vi "PAN_Send_InternalCmd.vi"(4 "timeout in ms (-1)":i32=30000, 6 "wait response":bool=TRUE, 7 "taskID":string, 8 "error in (no error)":errorcluster, 10 "command":string) -> (0 "error out":errorcluster, 2 "response":string)   [LabVIEW 2016]
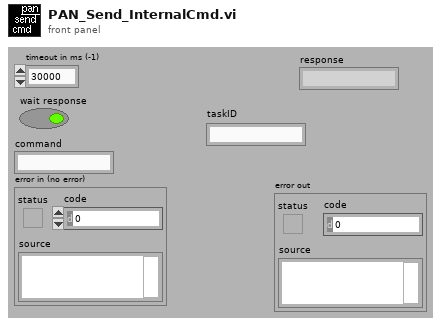
[diagram p1: front panel]
types:
  T1 = typedef "PAN_cmdStruct.ctl" = cluster{"command":string, "resp Q":refnum<queue>}
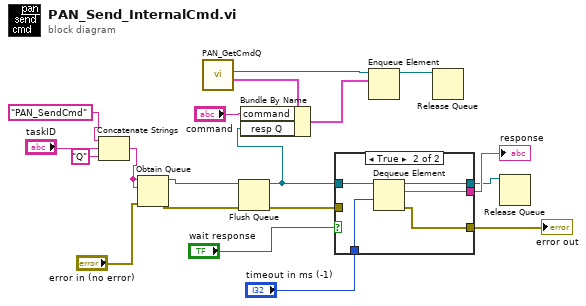
[diagram p0: block diagram]
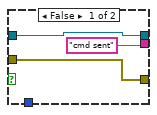
[diagram p2: hidden frame]
diagram:
  n1 = Concatenate Strings("PAN_SendCmd" ("name (unnamed)"), "taskID", "Q" ("string")) -> (w1:string)
  n2 = Obtain Queue(name (unnamed)=w1, element data type=w1, error in (no error)="error in (no error)") -> (queue out=w8:refnum<queue>, error out=w10:errorcluster)  [unwired: 2 in, 1 out]
  n3 = call "PAN_GetCmdQ.vi"() -> ("cmd struct"=w19:T1, "cmdQ"=w18:refnum<queue>)  [unwired: 10 out]
  n4 = Flush Queue(queue=w8, error in (no error)=w10) -> (queue out=w5:refnum<queue>, error out=w11:errorcluster)  [unwired: 1 out]
  n5 = Bundle By Name(cluster=w19, "command"="command", "resp Q"=w5) -> (w17:T1)
  n6 = case shown="True" "wait response" {
    tunnel: w5 -> [w20 w25]
    tunnel: "timeout in ms (-1)" -> [_ w27]
    tunnel: [w22 w26] -> w12
    tunnel: w11 -> [w22 _]
    tunnel: ["cmd sent" ("name (unnamed)") w24] -> w7
    tunnel: [w20 w23] -> w6
    frame False {
    }
    frame True {
      n7 = Dequeue Element(queue=w25, timeout in ms (-1)=w27) -> (queue out=w23:refnum<queue>, element=w24:string, error out=w26:errorcluster)  [unwired: 1 in, 1 out]
    }
  }
  "response" <- w7
  "error out" <- w12
  n8 = Enqueue Element(queue=w18, element=w17) -> (queue out=w16:refnum<queue>)  [unwired: 1 in, 3 out]
  n9 = Release Queue(queue=w16) -> ()  [unwired: 1 in, 4 out]
  n10 = Release Queue(queue=w6) -> ()  [unwired: 1 in, 4 out]
